vi "bitwise.vi"(7 "移位":i16=-4, 8 "置1":u8=240, 9 "索引":i32=37, 11 "数组":u8[](array[numeric])) -> (2 "y2":u8, 3 "y1":u8)   [LabVIEW 2012]
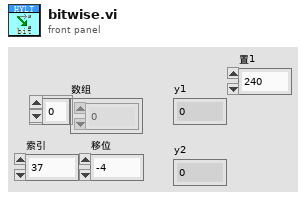
[diagram p1: front panel]
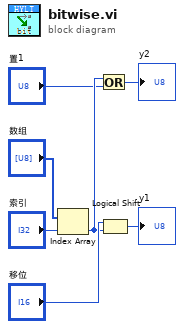
[diagram p0: block diagram]
diagram:
  n1 = Index Array(array="数组", index="索引") -> (element=w4:u8)
  n2 = Or(x=w4, y="置1") -> (x .or. y?=→"y2":u8)
  n3 = Logical Shift(y="移位", x=w4) -> (x << y=→"y1":u8)
